vi "Calculate.vi"(8 "error in (no error)":errorcluster, 10 "X (degrees)":dbl, 11 "AngleFunction in":refnum<class "LinearInterpolation.lvclass">) -> (0 "error out":errorcluster, 2 "AngleFunction(X)":dbl, 3 "AngleFunction out":refnum<class "LinearInterpolation.lvclass">)   [LabVIEW 2012, in "LinearInterpolation.lvclass"]
uses:
  LinearInterpolation.lvclass
panel:
  in  "Test Angles":dbl[](array[numeric])=[10.0, 20.0, 30.0, 40.0, 50.0, 60.0, 70.0, 80.0, 90.0, 100.0]
  in  "Test Values":dbl[](array[numeric])=[1.0, 2.0, 3.0, 4.0, 5.0, 6.0, 7.0, 8.0, 9.0, 10.0]
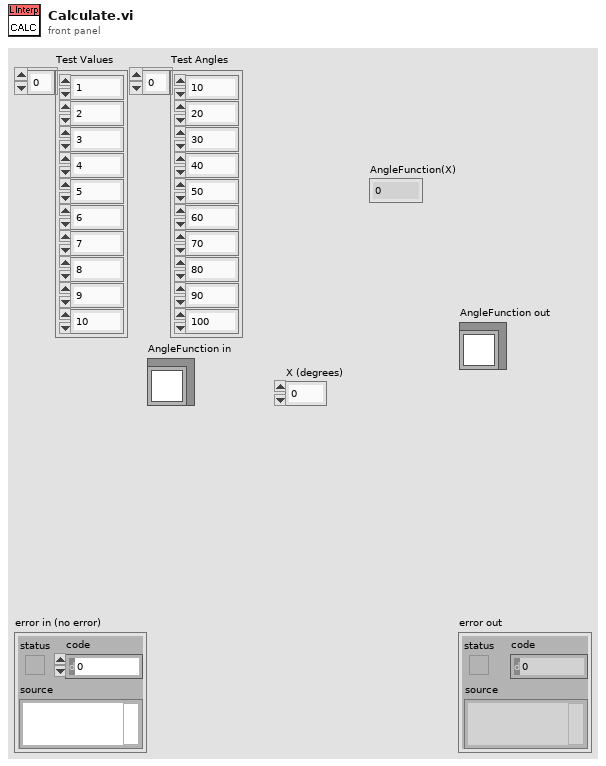
[diagram p1: front panel]
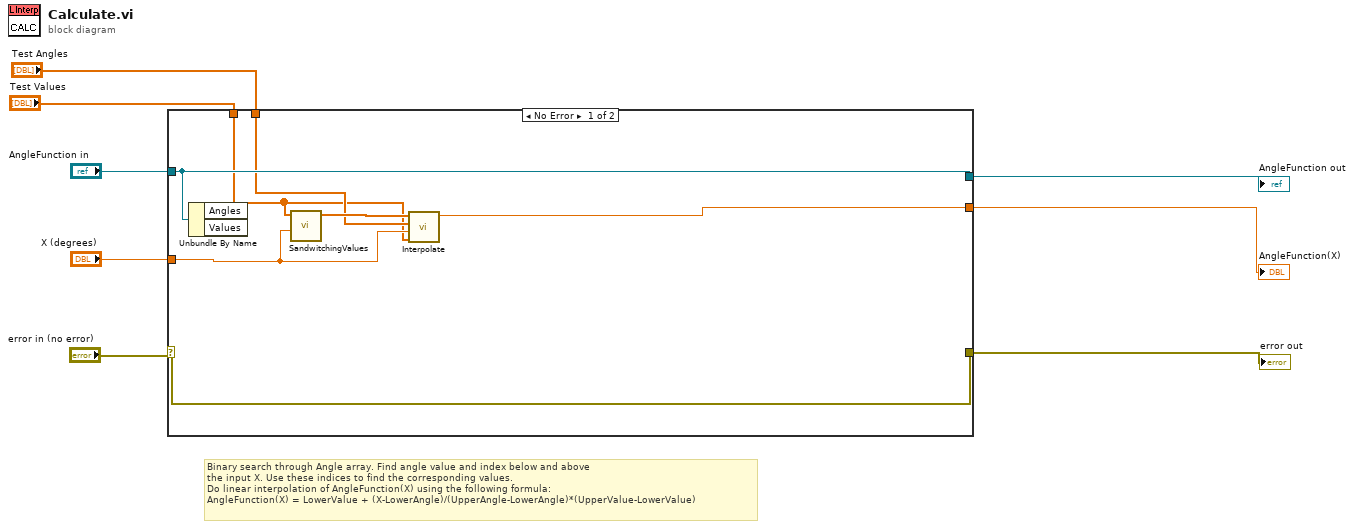
[diagram p0: block diagram]
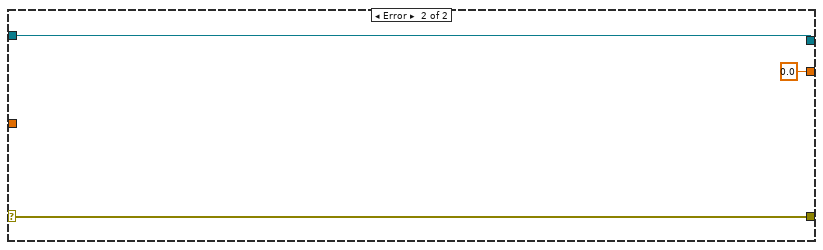
[diagram p2: hidden frame]
diagram:
  # "Binary search through Angle array. Find angle value and index below and above\nthe input X. Use these indices to find the corresponding values.\nDo linear interpolation of AngleFunction(X) using the following formula:\nAngleFunction(X) = LowerValue + (X-LowerAngle)/(UpperAngle-LowerAngle)*(UpperValue-LowerValue)"
  n1 = case shown="No Error" "error in (no error)" {
    selector: "error in (no error)" -> [w15 w17]
    tunnel: "AngleFunction in" -> [w14 w18]
    tunnel: "X (degrees)" -> [w11 _]
    tunnel: [w15 w17] -> w5
    tunnel: [w14 w18] -> w4
    tunnel: "Test Values" -> [w9 _]
    tunnel: "Test Angles" -> [w10 _]
    tunnel: [w13 0.0 ("InterpolatedValue")] -> w1
    frame No Error {
      n2 = Unbundle By Name(w14) -> ()  [unwired: 2 out]
      n3 = call "SandwitchingValues.vi"("DesiredAngle"=w11, "Angle Array"=w9) -> ("Angle Indexes"=w12:dbl[])  [unwired: 8 in]
      n4 = call "Interpolate.vi"("Angles"=w9, "DesiredAngle"=w11, "Values"=w10, "Indexes"=w12) -> ("InterpolatedValue"=w13:dbl)  [unwired: 7 in]
    }
    frame Error {
    }
  }
  "error out" <- w5
  "AngleFunction out" <- w4
  "AngleFunction(X)" <- w1
